vi "PresentSword.vi"(8 "Error In":errorcluster, 10 "Slide Refnum":refnum<vi>, 11 "Jedi in":refnum<class "Jedi.lvclass">) -> (0 "Error Out":errorcluster, 3 "Jedi out":refnum<class "Jedi.lvclass">)   [LabVIEW 2021, in "Jedi.lvclass"]
uses:
  Jedi.lvclass
  Jedi.lvclass/Jedi.ctl
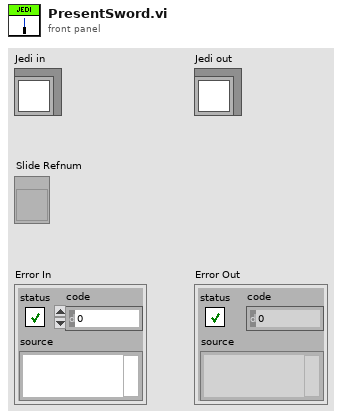
[diagram p1: front panel]
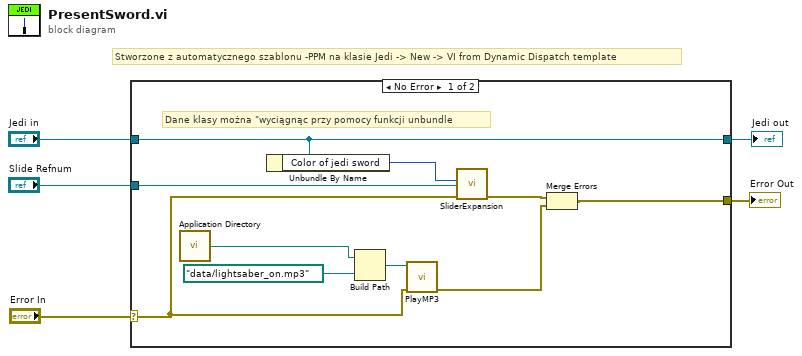
[diagram p0: block diagram]
diagram:
  # "Stworzone z automatycznego szablonu -PPM na klasie Jedi -> New -> VI from Dynamic Dispatch template"
  n1 = case shown="No Error" "Error In" {
    selector: "Error In" -> [w9 w17]
    tunnel: [w6 w17] -> w4
    tunnel: [w15 w16] -> w2
    tunnel: "Jedi in" -> [w15 w16]
    tunnel: "Slide Refnum" -> [w13 _]
    frame No Error {
      # "Dane klasy można \"wyciągnąc przy pomocy funkcji unbundle"
      n2 = call <vilib>:"Application Directory.vi"() -> ("Application Directory"=w12:path)
      n3 = Unbundle By Name(w15) -> ("Color of jedi sword"=w14:u32)
      n4 = Build Path(base path=w12, name or relative path=path "data/lightsaber_on.mp3") -> (appended path=w10:path)
      n5 = call "PlayMP3.vi"("Error In"=w9, "Path"=w10) -> ("Error out"=w7:errorcluster)  [unwired: 9 in]
      n6 = call "SliderExpansion.vi"("Error Out"=w9, "Slider color"=w14, "Slide Refnum"=w13) -> ("Error Out"=w8:errorcluster)  [unwired: 8 in]
      n7 = Merge Errors(w8, w7) -> (w6:errorcluster)
    }
    frame Error {
    }
  }
  "Error Out" <- w4
  "Jedi out" <- w2
